vi "Arcade Joystick Mapping.vi"() -> ()   [LabVIEW 2025]
doc: "This example shows how arcade joystick mapping controls motor outputs."
panel:
  out "Arcade Inputs":picture
  out "Left":dbl[][](graph)=[[0.0, -0.09999999999999998, -0.19999999999999996, -0.30000000000000004, -0.4, -0.5, -0.6000000000000001, -0.7000000000000001, -0.8, -0.9, -1.0, -1.0, -1.0, -1.0, -1.0, -1.0, -1.0, -1.0, -1.0, -1.0, -1.0], [0.09999999999999998, 0.0, -0.09999999999999998, -0.20000000000000007, -0.30000000000000004, -0.4, -0.5000000000000001, -0.6000000000000001, -0.7000000000000001, -0.8, -0.9, -0.9, -0.9, -0.9, -0.9, -0.9, -0.9, -0.9, -0.9, -0.9000000000000001, -1.0], [0.19999999999999996, 0.09999999999999998, 0.0, -0.10000000000000009, -0.20000000000000007, -0.30000000000000004, -0.40000000000000013, -0.5000000000000001, -0.6000000000000001, -0.7000000000000001, -0.8, -0.8, -0.8, -0.8, -0.8, -0.8, -0.8, -0.8, -0.8, -0.9000000000000001, -1.0], [0.30000000000000004, 0.20000000000000007, 0.10000000000000009, 0.0, -0.09999999999999998, -0.19999999999999996, -0.30000000000000004, -0.4, -0.5, -0.6, -0.7, -0.7, -0.7, -0.7, -0.7, -0.7, -0.7, -0.7000000000000002, -0.8, -0.9000000000000001, -1.0], [0.4, 0.30000000000000004, 0.20000000000000007, 0.09999999999999998, 0.0, -0.09999999999999998, -0.20000000000000007, -0.30000000000000004, -0.4, -0.5, -0.6, -0.6, -0.6, -0.6, -0.6, -0.6, -0.6000000000000001, -0.7000000000000002, -0.8, -0.9000000000000001, -1.0], [0.5, 0.4, 0.30000000000000004, 0.19999999999999996, 0.09999999999999998, 0.0, -0.10000000000000009, -0.20000000000000007, -0.30000000000000004, -0.4, -0.5, -0.5, -0.5, -0.5, -0.5, -0.5, -0.6000000000000001, -0.7000000000000002, -0.8, -0.9000000000000001, -1.0], [0.6000000000000001, 0.5000000000000001, 0.40000000000000013, 0.30000000000000004, 0.20000000000000007, 0.10000000000000009, 0.0, -0.09999999999999998, -0.19999999999999996, -0.29999999999999993, -0.3999999999999999, -0.3999999999999999, -0.3999999999999999, -0.3999999999999999, -0.40000000000000013, -0.5, -0.6000000000000001, -0.7000000000000002, -0.8, -0.9000000000000001, -1.0], [0.7000000000000001, 0.6000000000000001, 0.5000000000000001, 0.4, 0.30000000000000004, 0.20000000000000007, 0.09999999999999998, 0.0, -0.09999999999999998, -0.19999999999999996, -0.29999999999999993, -0.29999999999999993, -0.29999999999999993, -0.30000000000000004, -0.40000000000000013, -0.5, -0.6000000000000001, -0.7000000000000002, -0.8, -0.9000000000000001, -1.0], [0.8, 0.7000000000000001, 0.6000000000000001, 0.5, 0.4, 0.30000000000000004, 0.19999999999999996, 0.09999999999999998, 0.0, -0.09999999999999998, -0.19999999999999996, -0.19999999999999996, -0.20000000000000018, -0.30000000000000004, -0.40000000000000013, -0.5, -0.6000000000000001, -0.7000000000000002, -0.8, -0.9000000000000001, -1.0], [0.9, 0.8, 0.7000000000000001, 0.6, 0.5, 0.4, 0.29999999999999993, 0.19999999999999996, 0.09999999999999998, 0.0, -0.09999999999999998, -0.10000000000000009, -0.20000000000000018, -0.30000000000000004, -0.40000000000000013, -0.5, -0.6000000000000001, -0.7000000000000002, -0.8, -0.9000000000000001, -1.0], [1.0, 0.9, 0.8, 0.7, 0.6, 0.5, 0.3999999999999999, 0.29999999999999993, 0.19999999999999996, 0.09999999999999998, 0.0, -0.10000000000000009, -0.20000000000000018, -0.30000000000000004, -0.40000000000000013, -0.5, -0.6000000000000001, -0.7000000000000002, -0.8, -0.9000000000000001, -1.0], [1.0, 0.9, 0.8, 0.7, 0.6, 0.5, 0.3999999999999999, 0.29999999999999993, 0.19999999999999996, 0.10000000000000009, 0.10000000000000009, 0.0, -0.10000000000000009, -0.19999999999999996, -0.30000000000000004, -0.3999999999999999, -0.5, -0.6000000000000001, -0.7, -0.8, -0.8999999999999999], [1.0, 0.9, 0.8, 0.7, 0.6, 0.5, 0.3999999999999999, 0.29999999999999993, 0.20000000000000018, 0.20000000000000018, 0.20000000000000018, 0.10000000000000009, 0.0, -0.09999999999999987, -0.19999999999999996, -0.2999999999999998, -0.3999999999999999, -0.5, -0.5999999999999999, -0.7, -0.7999999999999998], [1.0, 0.9, 0.8, 0.7, 0.6, 0.5, 0.3999999999999999, 0.30000000000000004, 0.30000000000000004, 0.30000000000000004, 0.30000000000000004, 0.19999999999999996, 0.09999999999999987, 0.0, -0.10000000000000009, -0.19999999999999996, -0.30000000000000004, -0.40000000000000013, -0.5, -0.6000000000000001, -0.7], [1.0, 0.9, 0.8, 0.7, 0.6, 0.5, 0.40000000000000013, 0.40000000000000013, 0.40000000000000013, 0.40000000000000013, 0.40000000000000013, 0.30000000000000004, 0.19999999999999996, 0.10000000000000009, 0.0, -0.09999999999999987, -0.19999999999999996, -0.30000000000000004, -0.3999999999999999, -0.5, -0.5999999999999999], [1.0, 0.9, 0.8, 0.7, 0.6, 0.5, 0.5, 0.5, 0.5, 0.5, 0.5, 0.3999999999999999, 0.2999999999999998, 0.19999999999999996, 0.09999999999999987, 0.0, -0.10000000000000009, -0.20000000000000018, -0.30000000000000004, -0.40000000000000013, -0.5], [1.0, 0.9, 0.8, 0.7, 0.6000000000000001, 0.6000000000000001, 0.6000000000000001, 0.6000000000000001, 0.6000000000000001, 0.6000000000000001, 0.6000000000000001, 0.5, 0.3999999999999999, 0.30000000000000004, 0.19999999999999996, 0.10000000000000009, 0.0, -0.10000000000000009, -0.19999999999999996, -0.30000000000000004, -0.3999999999999999], [1.0, 0.9, 0.8, 0.7000000000000002, 0.7000000000000002, 0.7000000000000002, 0.7000000000000002, 0.7000000000000002, 0.7000000000000002, 0.7000000000000002, 0.7000000000000002, 0.6000000000000001, 0.5, 0.40000000000000013, 0.30000000000000004, 0.20000000000000018, 0.10000000000000009, 0.0, -0.09999999999999987, -0.19999999999999996, -0.2999999999999998], [1.0, 0.9, 0.8, 0.8, 0.8, 0.8, 0.8, 0.8, 0.8, 0.8, 0.8, 0.7, 0.5999999999999999, 0.5, 0.3999999999999999, 0.30000000000000004, 0.19999999999999996, 0.09999999999999987, 0.0, -0.10000000000000009, -0.19999999999999996], [1.0, 0.9000000000000001, 0.9000000000000001, 0.9000000000000001, 0.9000000000000001, 0.9000000000000001, 0.9000000000000001, 0.9000000000000001, 0.9000000000000001, 0.9000000000000001, 0.9000000000000001, 0.8, 0.7, 0.6000000000000001, 0.5, 0.40000000000000013, 0.30000000000000004, 0.19999999999999996, 0.10000000000000009, 0.0, -0.09999999999999987], [1.0, 1.0, 1.0, 1.0, 1.0, 1.0, 1.0, 1.0, 1.0, 1.0, 1.0, 0.8999999999999999, 0.7999999999999998, 0.7, 0.5999999999999999, 0.5, 0.3999999999999999, 0.2999999999999998, 0.19999999999999996, 0.09999999999999987, 0.0]]
  in  "Spin":bool
  in  "Sensitivity":dbl(slide) scale=0.0..1.0
  in  "Square Inputs":bool
  in  "Arcade Type":enum16{"Standard", "Button Spin", "Ratio Curve"}(ring)
  out "Right":dbl[][](graph)=[[-1.0, -1.0, -1.0, -1.0, -1.0, -1.0, -1.0, -1.0, -1.0, -1.0, -1.0, -0.8999999999999999, -0.7999999999999998, -0.7, -0.5999999999999999, -0.5, -0.3999999999999999, -0.2999999999999998, -0.19999999999999996, -0.09999999999999987, 0.0], [-1.0, -0.9, -0.9, -0.9, -0.9, -0.9, -0.9, -0.9, -0.9, -0.9, -0.9, -0.7999999999999999, -0.6999999999999998, -0.6, -0.4999999999999999, -0.4, -0.29999999999999993, -0.19999999999999984, -0.09999999999999998, 1.1102230246251565e-16, 0.09999999999999998], [-1.0, -0.9, -0.8, -0.8, -0.8, -0.8, -0.8, -0.8, -0.8, -0.8, -0.8, -0.7, -0.5999999999999999, -0.5, -0.3999999999999999, -0.30000000000000004, -0.19999999999999996, -0.09999999999999987, 0.0, 0.10000000000000009, 0.19999999999999996], [-1.0, -0.9, -0.8, -0.7, -0.7, -0.7, -0.7, -0.7, -0.7, -0.7, -0.7, -0.5999999999999999, -0.4999999999999998, -0.3999999999999999, -0.2999999999999998, -0.19999999999999996, -0.09999999999999987, 2.220446049250313e-16, 0.10000000000000009, 0.20000000000000018, 0.30000000000000004], [-1.0, -0.9, -0.8, -0.7, -0.6, -0.6, -0.6, -0.6, -0.6, -0.6, -0.6, -0.4999999999999999, -0.3999999999999998, -0.29999999999999993, -0.19999999999999984, -0.09999999999999998, 1.1102230246251565e-16, 0.1000000000000002, 0.20000000000000007, 0.30000000000000016, 0.4], [-1.0, -0.9, -0.8, -0.7, -0.6, -0.5, -0.5, -0.5, -0.5, -0.5, -0.5, -0.3999999999999999, -0.2999999999999998, -0.19999999999999996, -0.09999999999999987, 0.0, 0.10000000000000009, 0.20000000000000018, 0.30000000000000004, 0.40000000000000013, 0.5], [-1.0, -0.9, -0.8, -0.7, -0.6, -0.5, -0.3999999999999999, -0.3999999999999999, -0.3999999999999999, -0.3999999999999999, -0.3999999999999999, -0.2999999999999998, -0.19999999999999973, -0.09999999999999987, 2.220446049250313e-16, 0.10000000000000009, 0.20000000000000018, 0.30000000000000027, 0.40000000000000013, 0.5000000000000002, 0.6000000000000001], [-1.0, -0.9, -0.8, -0.7, -0.6, -0.5, -0.3999999999999999, -0.29999999999999993, -0.29999999999999993, -0.29999999999999993, -0.29999999999999993, -0.19999999999999984, -0.09999999999999976, 1.1102230246251565e-16, 0.1000000000000002, 0.20000000000000007, 0.30000000000000016, 0.40000000000000024, 0.5000000000000001, 0.6000000000000002, 0.7000000000000001], [-1.0, -0.9, -0.8, -0.7, -0.6, -0.5, -0.3999999999999999, -0.29999999999999993, -0.19999999999999996, -0.19999999999999996, -0.19999999999999996, -0.09999999999999987, 2.220446049250313e-16, 0.10000000000000009, 0.20000000000000018, 0.30000000000000004, 0.40000000000000013, 0.5000000000000002, 0.6000000000000001, 0.7000000000000002, 0.8], [-1.0, -0.9, -0.8, -0.7, -0.6, -0.5, -0.3999999999999999, -0.29999999999999993, -0.19999999999999996, -0.09999999999999998, -0.09999999999999998, 1.1102230246251565e-16, 0.1000000000000002, 0.20000000000000007, 0.30000000000000016, 0.4, 0.5000000000000001, 0.6000000000000002, 0.7000000000000001, 0.8000000000000002, 0.9], [-1.0, -0.9, -0.8, -0.7, -0.6, -0.5, -0.3999999999999999, -0.29999999999999993, -0.19999999999999996, -0.09999999999999998, 0.0, 0.10000000000000009, 0.20000000000000018, 0.30000000000000004, 0.40000000000000013, 0.5, 0.6000000000000001, 0.7000000000000002, 0.8, 0.9000000000000001, 1.0], [-0.8999999999999999, -0.7999999999999999, -0.7, -0.5999999999999999, -0.4999999999999999, -0.3999999999999999, -0.2999999999999998, -0.19999999999999984, -0.09999999999999987, 1.1102230246251565e-16, 0.10000000000000009, 0.10000000000000009, 0.20000000000000018, 0.30000000000000004, 0.40000000000000013, 0.5, 0.6000000000000001, 0.7000000000000002, 0.8, 0.9000000000000001, 1.0], [-0.7999999999999998, -0.6999999999999998, -0.5999999999999999, -0.4999999999999998, -0.3999999999999998, -0.2999999999999998, -0.19999999999999973, -0.09999999999999976, 2.220446049250313e-16, 0.1000000000000002, 0.20000000000000018, 0.20000000000000018, 0.20000000000000018, 0.30000000000000004, 0.40000000000000013, 0.5, 0.6000000000000001, 0.7000000000000002, 0.8, 0.9000000000000001, 1.0], [-0.7, -0.6, -0.5, -0.3999999999999999, -0.29999999999999993, -0.19999999999999996, -0.09999999999999987, 1.1102230246251565e-16, 0.10000000000000009, 0.20000000000000007, 0.30000000000000004, 0.30000000000000004, 0.30000000000000004, 0.30000000000000004, 0.40000000000000013, 0.5, 0.6000000000000001, 0.7000000000000002, 0.8, 0.9000000000000001, 1.0], [-0.5999999999999999, -0.4999999999999999, -0.3999999999999999, -0.2999999999999998, -0.19999999999999984, -0.09999999999999987, 2.220446049250313e-16, 0.1000000000000002, 0.20000000000000018, 0.30000000000000016, 0.40000000000000013, 0.40000000000000013, 0.40000000000000013, 0.40000000000000013, 0.40000000000000013, 0.5, 0.6000000000000001, 0.7000000000000002, 0.8, 0.9000000000000001, 1.0], [-0.5, -0.4, -0.30000000000000004, -0.19999999999999996, -0.09999999999999998, 0.0, 0.10000000000000009, 0.20000000000000007, 0.30000000000000004, 0.4, 0.5, 0.5, 0.5, 0.5, 0.5, 0.5, 0.6000000000000001, 0.7000000000000002, 0.8, 0.9000000000000001, 1.0], [-0.3999999999999999, -0.29999999999999993, -0.19999999999999996, -0.09999999999999987, 1.1102230246251565e-16, 0.10000000000000009, 0.20000000000000018, 0.30000000000000016, 0.40000000000000013, 0.5000000000000001, 0.6000000000000001, 0.6000000000000001, 0.6000000000000001, 0.6000000000000001, 0.6000000000000001, 0.6000000000000001, 0.6000000000000001, 0.7000000000000002, 0.8, 0.9000000000000001, 1.0], [-0.2999999999999998, -0.19999999999999984, -0.09999999999999987, 2.220446049250313e-16, 0.1000000000000002, 0.20000000000000018, 0.30000000000000027, 0.40000000000000024, 0.5000000000000002, 0.6000000000000002, 0.7000000000000002, 0.7000000000000002, 0.7000000000000002, 0.7000000000000002, 0.7000000000000002, 0.7000000000000002, 0.7000000000000002, 0.7000000000000002, 0.8, 0.9000000000000001, 1.0], [-0.19999999999999996, -0.09999999999999998, 0.0, 0.10000000000000009, 0.20000000000000007, 0.30000000000000004, 0.40000000000000013, 0.5000000000000001, 0.6000000000000001, 0.7000000000000001, 0.8, 0.8, 0.8, 0.8, 0.8, 0.8, 0.8, 0.8, 0.8, 0.9000000000000001, 1.0], [-0.09999999999999987, 1.1102230246251565e-16, 0.10000000000000009, 0.20000000000000018, 0.30000000000000016, 0.40000000000000013, 0.5000000000000002, 0.6000000000000002, 0.7000000000000002, 0.8000000000000002, 0.9000000000000001, 0.9000000000000001, 0.9000000000000001, 0.9000000000000001, 0.9000000000000001, 0.9000000000000001, 0.9000000000000001, 0.9000000000000001, 0.9000000000000001, 0.9000000000000001, 1.0], [0.0, 0.09999999999999998, 0.19999999999999996, 0.30000000000000004, 0.4, 0.5, 0.6000000000000001, 0.7000000000000001, 0.8, 0.9, 1.0, 1.0, 1.0, 1.0, 1.0, 1.0, 1.0, 1.0, 1.0, 1.0, 1.0]]
  out "Right Power":dbl(knob) scale=-1.0..1.0
  out "Left Power":dbl(knob) scale=1.0..-1.0
  # "Joystick Conventions:\nHID joystick conventions use -1 for forward and left and 1 for back and right,\n\nExplore the different types and options for arcade joystick control."
  # "Algorithm Setup"
  # "Axis Inputs"
  # "Click or drag circle"
  # "Front (-1)"
  # "Left (-1)"
  # "Right (1)"
  # "Back (1)"
  # "Motor Power"
  # "Color Legend"
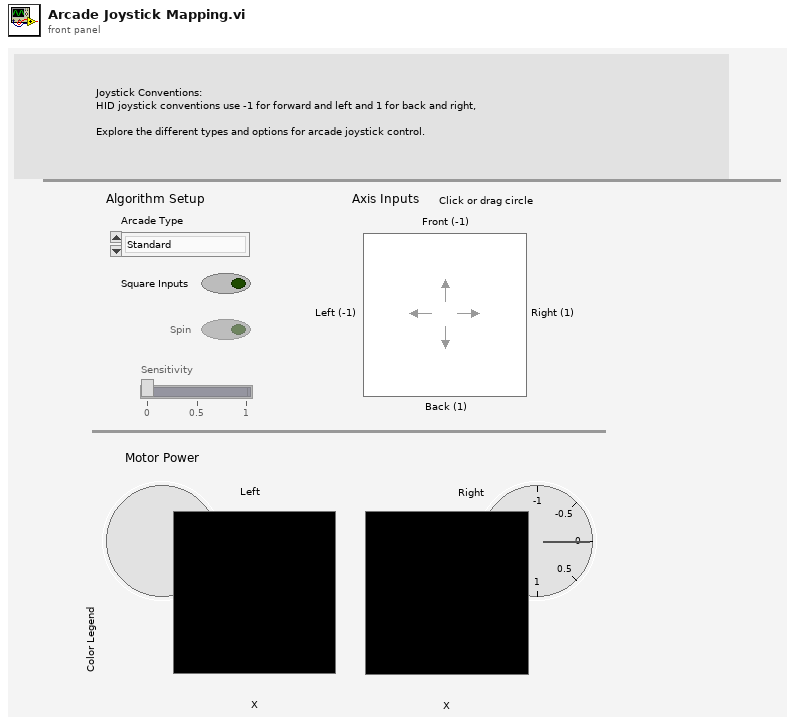
[diagram p1: front panel]
types:
  T1 = cluster{"Disabled":enum8{"Enabled", "Disabled", "Disabled and Grayed Out"}, "Disabled 2":enum8{"Enabled", "Disabled", "Disabled and Grayed Out"}, "Disabled 3":enum8{"Enabled", "Disabled", "Disabled and Grayed Out"}}[]
  T2 = typedef "LVPositionTypeDef.ctl" = cluster{"Left":i32, "Top":i32}
  T3 = typedef "LVBoundsTypeDef.ctl" = cluster{"Width":u32, "Height":u32}
  T4 = typedef "LVMouseTypeDef.ctl" = cluster{"Mouse Position":cluster{"X":i32, "Y":i32}, "Mouse Modifiers":cluster{"Button Down":bool, "Shift Mod":bool, "Menu Mod":bool, "Option Mod":bool}}
  T5 = cluster{"Disabled":enum8{"Enabled", "Disabled", "Disabled and Grayed Out"}, "Disabled 2":enum8{"Enabled", "Disabled", "Disabled and Grayed Out"}, "Disabled 3":enum8{"Enabled", "Disabled", "Disabled and Grayed Out"}}
  T6 = enum8{"Enabled", "Disabled", "Disabled and Grayed Out"}
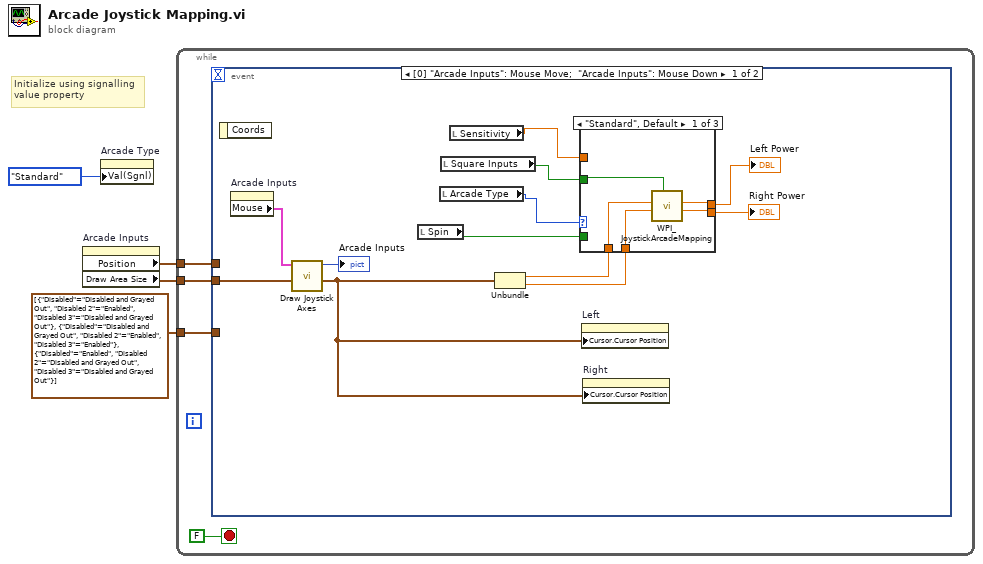
[diagram p0: block diagram]
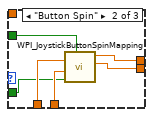
[diagram p2: hidden frame]
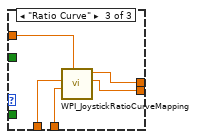
[diagram p3: hidden frame]
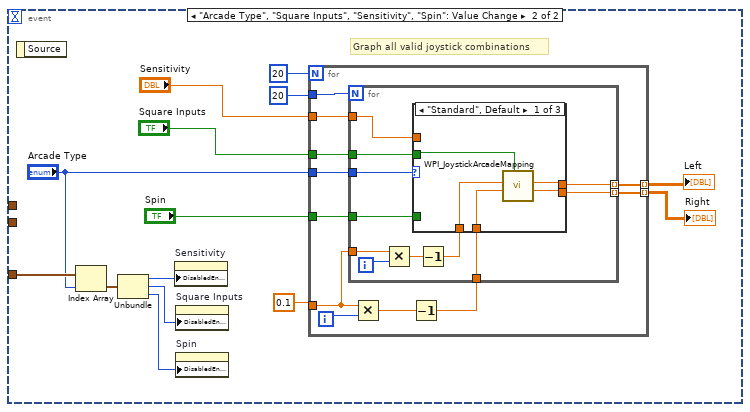
[diagram p4: hidden frame]
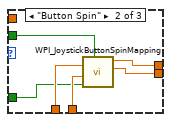
[diagram p5: hidden frame]
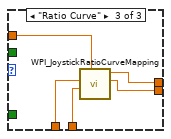
[diagram p6: hidden frame]
diagram:
  # "Initialize using signalling\nvalue property"
  n1 = property on="Arcade Inputs" class="Pict"() -> ("Position"=w1:T2, "Draw Area Size"=w2:T3)  [unwired: 2 in, 2 out]
  n2 = property on="Arcade Type" class="Enum (strict)"("Val(Sgnl)"=enum16{"Standard", "Button Spin", "Ratio Curve"}."Standard" ("Value (Signaling)")) -> ()  [unwired: 2 in, 2 out]
  n3 = while {
    tunnel: T1 [{"Disabled"=enum."Disabled and Grayed Out", "Disabled 2"=enum."Enabled", "Disabled 3"=enum."Disabled and Grayed Out"}, {"Disabled"=enum."Disabled and Grayed Out", "Disabled 2"=enum."Enabled", "Disabled 3"=enum."Enabled"}, {"Disabled"=enum."Enabled", "Disabled 2"=enum."Disabled and Grayed Out", "Disabled 3"=enum."Disabled and Grayed Out"}] -> [w7]
    tunnel: w2 -> [w6]
    tunnel: w1 -> [w5]
    stop <- FALSE stop-if-true
    n4 = event shown="[0] \"Arcade Inputs\": Mouse Move;  \"Arcade Inputs\": Mouse Down" {
      selector: _ -> [_ _]
      dyn-events: _ -> [_ _]
      timeout: _ -> [_ _]
      tunnel: w7 -> [_ w50]
      tunnel: w6 -> [w19 _]
      tunnel: w5 -> [_ _]
      event "Arcade Inputs": Mouse Move; "Arcade Inputs": Mouse Down {
        n5 = event-data() -> ()  [unwired: 1 in, 1 out]
        n6 = property on="Arcade Inputs" class="Pict"() -> ("Mouse"=w9:T4)  [unwired: 2 in, 2 out]
        n7 = call "Draw Joystick Axes.vi"("Size"=w19, "Mouse"=w9) -> ("JS Coords"=w10:cluster{"X":dbl, "Y":dbl}, "Arcade Inputs"=→"Arcade Inputs":picture)  [unwired: 8 in]
        n8 = local read "Spin"() -> (w13:bool)
        n9 = local read "Arcade Type"() -> (w14:enum16{"Standard", "Button Spin", "Ratio Curve"})
        n10 = local read "Square Inputs"() -> (w15:bool)
        n11 = local read "Sensitivity"() -> (w16:dbl)
        n12 = Unbundle(w10) -> ("X"=w12:dbl, "Y"=w11:dbl)
        n13 = case shown="\"Standard\", Default" w14 {
          tunnel: w12 -> [w24 w31 w34]
          tunnel: w11 -> [w23 w30 w33]
          tunnel: [w22 w29 w36] -> w17
          tunnel: [w21 w28 w35] -> w18
          tunnel: w15 -> [w25 w27 _]
          tunnel: w13 -> [_ w26 _]
          tunnel: w16 -> [_ _ w32]
          frame "Standard", Default {
            n14 = call <vilib>:"WPI_JoystickArcadeMapping.vi"("Square Inputs"=w25, "Y axis value"=w23, "X axis value"=w24) -> ("Right Motor Value"=w21:dbl, "Left Motor Value"=w22:dbl)  [unwired: 7 in]
          }
          frame "Button Spin" {
            n15 = call <vilib>:"WPI_JoystickButtonSpinMapping.vi"("Square Inputs"=w27, "Spin?"=w26, "Y axis value"=w30, "X axis value"=w31) -> ("Right Motor Value"=w28:dbl, "Left Motor Value"=w29:dbl)  [unwired: 6 in]
          }
          frame "Ratio Curve" {
            n16 = call <vilib>:"WPI_JoystickRatioCurveMapping.vi"("Sensitivity"=w32, "Y axis value (Speed)"=w33, "X axis value (Curve)"=w34) -> ("Right Motor Value"=w35:dbl, "Left Motor Value"=w36:dbl)  [unwired: 7 in]
          }
        }
        "Left Power" <- w17
        "Right Power" <- w18
        n17 = property on="Left" class="IntGraph (strict)"("Cursor.Cursor Position"=w10) -> ()  [unwired: 2 in, 2 out]
        n18 = property on="Right" class="IntGraph (strict)"("Cursor.Cursor Position"=w10) -> ()  [unwired: 2 in, 2 out]
      }
      event "Arcade Type", "Square Inputs", "Sensitivity", "Spin": Value Change {
        # "Graph all valid joystick combinations"
        n19 = event-data() -> ()  [unwired: 1 in, 1 out]
        n20 = Index Array(array=w50, index="Arcade Type") -> (element=w46:T5)
        n21 = Unbundle(w46) -> ("Disabled"=w47:T6, "Disabled 2"=w48:T6, "Disabled 3"=w49:T6)
        n22 = property on="Sensitivity" class="Slide (strict)"("DisabledEnum"=w47) -> ()  [unwired: 2 in, 2 out]
        n23 = property on="Square Inputs" class="Bool (strict)"("DisabledEnum"=w48) -> ()  [unwired: 2 in, 2 out]
        n24 = property on="Spin" class="Bool (strict)"("DisabledEnum"=w49) -> ()  [unwired: 2 in, 2 out]
        n25 = for {
          N: 20 -> [_]
          tunnel: 0.1 -> [w60]
          tunnel: [w58] -> w44 mode=indexing
          tunnel: [w57] -> w45 mode=indexing
          tunnel: 20 -> [w56]
          tunnel: "Square Inputs" -> [w54]
          tunnel: "Arcade Type" -> [w53]
          tunnel: "Spin" -> [w52]
          tunnel: "Sensitivity" -> [w51]
          i -> [w61]
          n26 = Multiply(x=w60, y=w61) -> (x*y=w59:dbl)
          n27 = Decrement(x=w59) -> (x-1=w55:dbl)
          n28 = for {
            N: w56 -> [_]
            tunnel: w60 -> [w72]
            tunnel: w55 -> [w68]
            tunnel: [w67] -> w58 mode=indexing
            tunnel: [w66] -> w57 mode=indexing
            tunnel: w54 -> [w65]
            tunnel: w53 -> [w64]
            tunnel: w52 -> [w63]
            tunnel: w51 -> [w62]
            i -> [w71]
            n29 = Multiply(x=w72, y=w71) -> (x*y=w70:dbl)
            n30 = Decrement(x=w70) -> (x-1=w69:dbl)
            n31 = case shown="\"Standard\", Default" w64 {
              tunnel: w69 -> [w76 w83 w86]
              tunnel: w68 -> [w75 w82 w85]
              tunnel: [w74 w81 w88] -> w67
              tunnel: [w73 w80 w87] -> w66
              tunnel: w65 -> [w77 w79 _]
              tunnel: w63 -> [_ w78 _]
              tunnel: w62 -> [_ _ w84]
              frame "Standard", Default {
                n32 = call <vilib>:"WPI_JoystickArcadeMapping.vi"("Square Inputs"=w77, "Y axis value"=w75, "X axis value"=w76) -> ("Right Motor Value"=w73:dbl, "Left Motor Value"=w74:dbl)  [unwired: 7 in]
              }
              frame "Button Spin" {
                n33 = call <vilib>:"WPI_JoystickButtonSpinMapping.vi"("Square Inputs"=w79, "Spin?"=w78, "Y axis value"=w82, "X axis value"=w83) -> ("Right Motor Value"=w80:dbl, "Left Motor Value"=w81:dbl)  [unwired: 6 in]
              }
              frame "Ratio Curve" {
                n34 = call <vilib>:"WPI_JoystickRatioCurveMapping.vi"("Sensitivity"=w84, "Y axis value (Speed)"=w85, "X axis value (Curve)"=w86) -> ("Right Motor Value"=w87:dbl, "Left Motor Value"=w88:dbl)  [unwired: 7 in]
              }
            }
          }
        }
        "Right" <- w45
        "Left" <- w44
      }
    }
  }
